vi "Day06-2.vi"() -> ()   [LabVIEW 2021]
panel:
  out "Total fish":u64
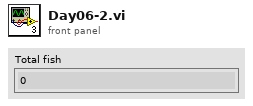
[diagram p1: front panel]
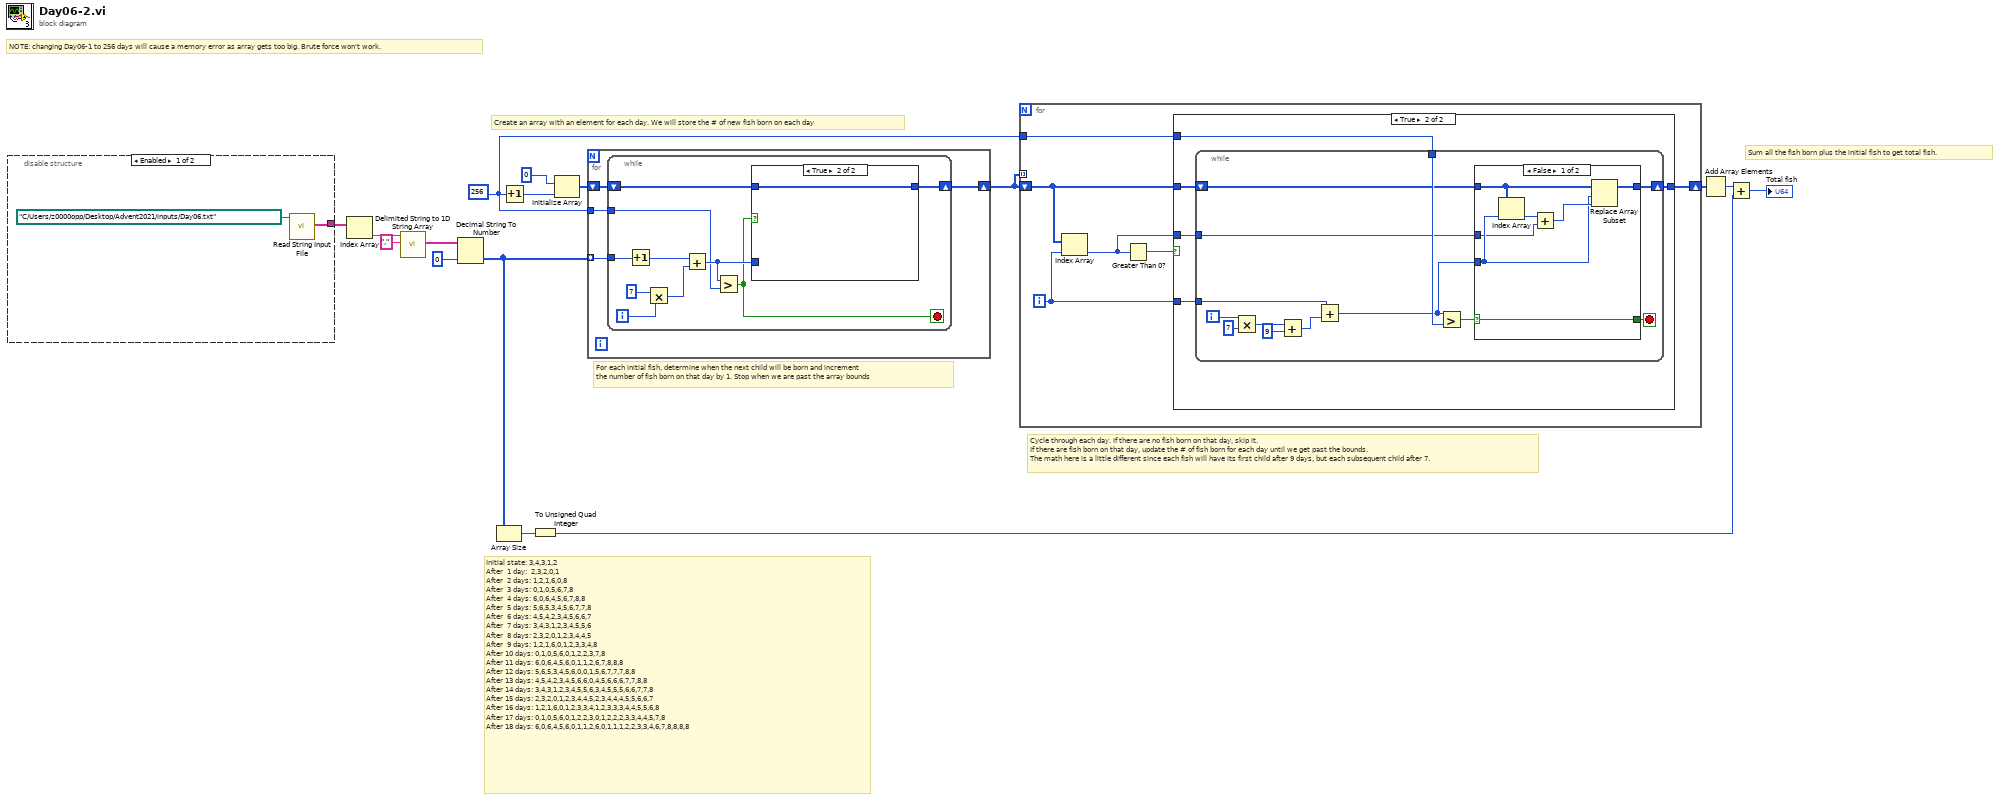
[diagram p0: block diagram]
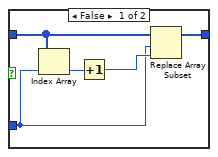
[diagram p4: hidden frame]
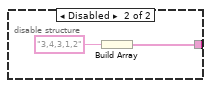
[diagram p5: hidden frame]
diagram:
  w8 = 256
  # "Sum all the fish born plus the initial fish to get total fish."
  # "Cycle through each day. If there are no fish born on that day, skip it.\nIf there are fish born on that day, update the # of fish born for each day until we get past the bounds.\nThe math here is a little different since each fish will have its first child after 9 days, but each subsequent child after 7."
  # "For each initial fish, determine when the next child will be born and increment\nthe number of fish born on that day by 1. Stop when we are past the array bounds"
  # "Create an array with an element for each day. We will store the # of new fish born on each day"
  # "Initial state: 3,4,3,1,2\nAfter  1 day:  2,3,2,0,1\nAfter  2 days: 1,2,1,6,0,8\nAfter  3 days: 0,1,0,5,6,7,8\nAfter  4 days: 6,0,6,4,5,6,7,8,8\nAfter  5 days: 5,6,5,3,4,5,6,7,7,8\nAfter  6 days: 4,5,4,2,3,4,5,6,6,7\nAfter  7 days: 3,4,3,1,2,3,4,5,5,6\nAfter  8 days: 2,3,2,0,1,2,3,4,4,5\nAfter  9 days: 1,2,1,6,0,1,2,3,3,4,8\nAfter 10 days: 0,1,0,5,6,0,1,2,2,3,7,8\nAfter 11 days: 6,0,6,4,5,6,0,1,1,2,6,7,8,8,8\nAfter 12 days: 5,6,5,3,4,5,6,0,0,1,5,6,7,7,7,8,8\nAfter 13 days: 4,5,4,2,3,4,5,6,6,0,4,5,6,6,6,7,7,8,8\nAfter 14 days: 3,4,3,1,2,3,4,5,5,6,3,4,5,5,5,6,6,7,7,8\nAfter 15 days: 2,3,2,0,1,2,3,4,4,5,2,3,4,4,4,5,5,6,6,7\nAfter 16 days: 1,2,1,6,0,1,2,3,3,4,1,2,3,3,3,4,4,5,5,6,8\nAfter 17 days: 0,1,0,5,6,0,1,2,2,3,0,1,2,2,2,3,3,4,4,5,7,8\nAfter 18 days: 6,0,6,4,5,6,0,1,1,2,6,0,1,1,1,2,2,3,3,4,6,7,8,8,8,8"
  # "NOTE: changing Day06-1 to 256 days will cause a memory error as array gets too big. Brute force won't work."
  n1 = disable-structure shown="Enabled" {
    disable-tunnel: [w17 w19] -> w15
    frame Enabled {
      n2 = call "Read String Input File.vi"("file path (dialog if empty)"=path "C:/Users/z0000opp/Desktop/Advent2021/inputs/Day06.txt") -> ("input values"=w17:string[])  [unwired: 10 in]
    }
    frame Disabled {
      n3 = Build Array("3,4,3,1,2") -> (w19:string[])
    }
  }
  n4 = Index Array(array=w15) -> (element=w14:string)  [unwired: 1 in]
  n5 = call <vilib>:"Delimited String to 1D String Array.vi"("delimiter"=",", "delimited string"=w14) -> ("string array"=w16:string[])  [unwired: 9 in]
  n6 = Decimal String To Number(string=w16, default (0L)=0) -> (number=w5:i32[])  [unwired: 1 in, 1 out]
  n7 = Array Size(array=w5) -> (size(s)=w4:i32)
  n8 = Increment(x=w8) -> (x+1=w10:i32)
  n9 = To Unsigned Quad Integer(1:w4) -> (0:w1:u64)
  n10 = Initialize Array(u64 0 ("element"), w10) -> (w9:u64[])
  n11 = for {
    tunnel: w5 -> [w24] mode=indexing
    shift-right: [w21] -> w2
    shift-left: w9 -> [w23]
    tunnel: w8 -> [w22]
    n12 = while {
      tunnel: w24 -> [w26]
      shift-right: [w33] -> w21
      shift-left: w23 -> [w34]
      tunnel: w22 -> [w28]
      i -> [w32]
      stop <- w27 stop-if-true
      n13 = Increment(x=w26) -> (x+1=w25:i32)
      n14 = Multiply(x=7, y=w32) -> (x*y=w30:i32)
      n15 = Add(x=w25, y=w30) -> (x+y=w29:i32)
      n16 = Greater?(x=w29, y=w28) -> (0:w27:bool)
      n17 = case shown="True" w27 {
        tunnel: w34 -> [w38 w40]
        tunnel: [w36 w40] -> w33
        tunnel: w29 -> [w35 _]
        frame False {
          n18 = Index Array(array=w38, index=w35) -> (element=w39:u64)
          n19 = Increment(x=w39) -> (x+1=w37:u64)
          n20 = Replace Array Subset(array=w38, new element=w37, index=w35) -> (w36:u64[])
        }
        frame True {
        }
      }
    }
  }
  n21 = for {
    shift-right: [w45] -> w7
    shift-left: w2 -> [w43]
    tunnel: w8 -> [w44]
    tunnel: w2 -> [_] mode=indexing
    i -> [w42]
    n22 = Index Array(array=w43, index=w42) -> (element=w41:u64)
    n23 = Greater Than 0?(x=w41) -> (x > 0?=w46:bool)
    n24 = case shown="True" w46 {
      tunnel: w43 -> [w47 w52]
      tunnel: [w47 w51] -> w45
      tunnel: w41 -> [_ w48]
      tunnel: w42 -> [_ w50]
      tunnel: w44 -> [_ w49]
      frame False {
      }
      frame True {
        n25 = while {
          shift-right: [w62] -> w51
          shift-left: w52 -> [w63]
          tunnel: w50 -> [w65]
          tunnel: w49 -> [w64]
          tunnel: w48 -> [w60]
          i -> [w59]
          stop <- w53 stop-if-true
          n26 = Multiply(x=w59, y=7) -> (x*y=w55:i32)
          n27 = Add(x=w55, y=9) -> (x+y=w58:i32)
          n28 = Add(x=w65, y=w58) -> (x+y=w61:i32)
          n29 = Greater?(x=w61, y=w64) -> (0:w54:bool)
          n30 = case shown="False" w54 {
            selector: w54 -> [w66 w73]
            tunnel: w63 -> [w71 w74]
            tunnel: [w69 w74] -> w62
            tunnel: w61 -> [w68 _]
            tunnel: w60 -> [w67 _]
            tunnel: [w66 w73] -> w53
            frame False {
              n31 = Index Array(array=w71, index=w68) -> (element=w72:u64)
              n32 = Add(x=w72, y=w67) -> (x+y=w70:u64)
              n33 = Replace Array Subset(array=w71, new element=w70, index=w68) -> (w69:u64[])
            }
            frame True {
            }
          }
        }
      }
    }
  }
  n34 = Add Array Elements(numeric array=w7) -> (sum=w6:u64)
  n35 = Add(x=w6, y=w1) -> (x+y=→"Total fish":u64)
